vi "Unpack string.vi"(8 "error in (no error)":errorcluster, 11 "Python Toolkit in":refnum<class "Python Toolkit.lvclass">) -> (0 "error out":errorcluster, 2 "Value":string, 3 "Python Toolkit out":refnum<class "Python Toolkit.lvclass">)   [LabVIEW 2018, in "Python Toolkit.lvclass"]
doc: "Get the string returned by a python function"
uses:
  Python Toolkit.lvclass
  Python Toolkit.lvclass/Python Toolkit.ctl
  <vilib>/Enthought/Python Integration Toolkit/api/Unpack String.vi
  <vilib>/Enthought/Python Integration Toolkit/Python Integration Toolkit.lvlib
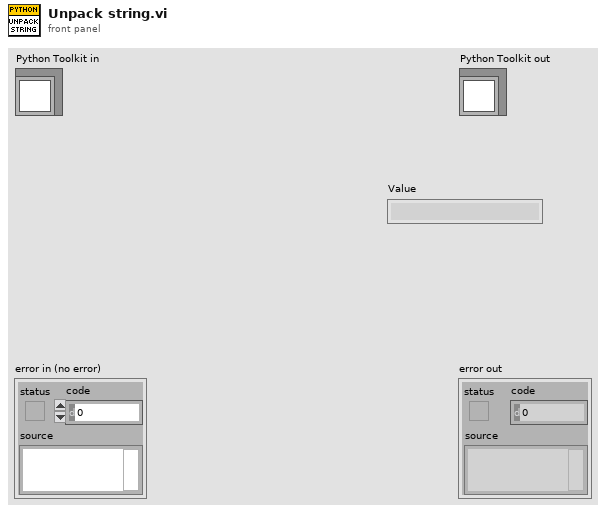
[diagram p1: front panel]
types:
  T1 = typedef "Python Integration Toolkit.lvlib/Session ID.ctl" = u64
  T2 = typedef "Python Integration Toolkit.lvlib/Python Objects.ctl" = variant
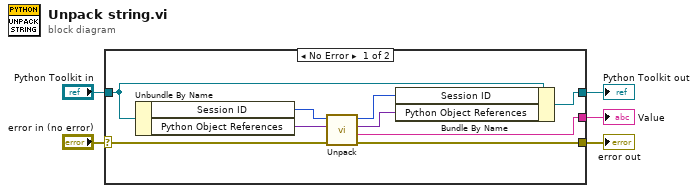
[diagram p0: block diagram]
diagram:
  n1 = case shown="No Error" "error in (no error)" {
    selector: "error in (no error)" -> [w14 w16]
    tunnel: [w13 w16] -> w4
    tunnel: [w9 w15] -> w2
    tunnel: "Python Toolkit in" -> [w10 w15]
    tunnel: [w6 _] -> w1
    frame No Error {
      n2 = Unbundle By Name(w10) -> ("Session ID"=w11:T1, "Python Object References"=w12:T2)
      n3 = call-poly <vilib>:"Unpack.vi"("error in (no error)"=w14, "Python Object References In"=w12, "Session ID"=w11) -> ("error out"=w13:errorcluster, "Value"=w6:string, "Python Object References Out"=w7:T2, "Session ID out"=w8:T1)  [unwired: 5 in]
      n4 = Bundle By Name(cluster=w10, "Session ID"=w8, "Python Object References"=w7) -> (w9:refnum<class "Python Toolkit.lvclass">)
    }
    frame Error {
    }
  }
  "error out" <- w4
  "Python Toolkit out" <- w2
  "Value" <- w1
